vi "Reorder cluster elements v1.2.vi"(8 "error in (no error)":errorcluster, 10 "Reference Variant":variant, 11 "Data Variant":variant) -> (0 "error out":errorcluster, 1 "Reference key names":string[](array[string]), 2 "Ordered VCluster":variant, 3 "Queried key names":string[](array[string]))   [LabVIEW 2015]
uses:
  <vilib>/Utility/Data Type/NI_Data Type.lvlib
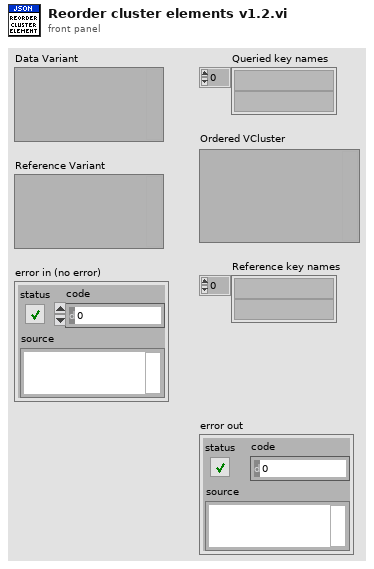
[diagram p1: front panel]
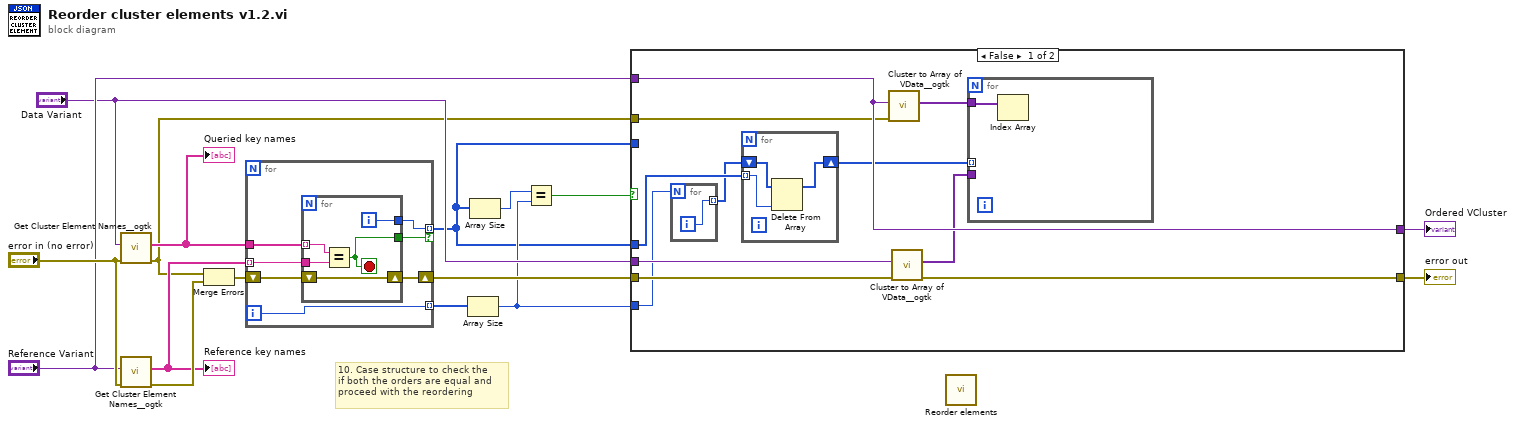
[diagram p0: block diagram]
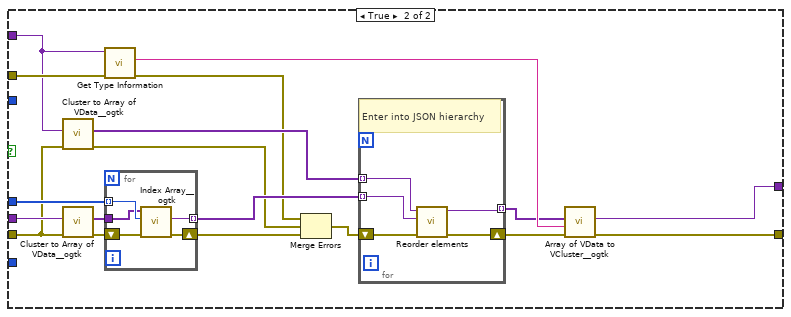
[diagram p2: hidden frame]
diagram:
  # "10. Case structure to check the\nif both the orders are equal and \nproceed with the reordering"
  n1 = call <userlib>:"Get Cluster Element Names__ogtk.vi"("error in (no error)"="error in (no error)", "Cluster"="Data Variant") -> ("error out"=w7:errorcluster, "Element Names"=w13:string[])  [unwired: 8 in]
  "Queried key names" <- w13
  n2 = call <userlib>:"Get Cluster Element Names__ogtk.vi"("error in (no error)"="error in (no error)", "Cluster"="Reference Variant") -> ("error out"=w14:errorcluster, "Element Names"=w12:string[])  [unwired: 8 in]
  "Reference key names" <- w12
  n3 = Merge Errors(w7, w14) -> (w15:errorcluster)
  n4 = for {
    tunnel: w12 -> [w22] mode=indexing
    tunnel: w13 -> [w23]
    tunnel: [w21] -> w1 mode=indexing if=w17
    shift-right: [w19] -> w16
    shift-left: w15 -> [w20]
    tunnel: [w18] -> w3 mode=indexing
    i -> [w18]
    n5 = for {
      tunnel: w23 -> [w28] mode=indexing
      tunnel: w22 -> [w27]
      tunnel: [w26] -> w21
      shift-right: [w25] -> w19
      shift-left: w20 -> [w25]
      tunnel: [w24] -> w17
      i -> [w26]
      stop <- w24 stop-if-true
      n6 = Equal?(x=w28, y=w27) -> (x = y?=w24:bool)
    }
  }
  n7 = Array Size(array=w3) -> (size(s)=w2:i32)
  n8 = Array Size(array=w1) -> (size(s)=w5:i32)
  n9 = Equal?(x=w5, y=w2) -> (x = y?=w4:bool)
  n10 = case shown="False" w4 {
    tunnel: w1 -> [w33 w62]
    tunnel: w16 -> [w36 w54]
    tunnel: "Reference Variant" -> [w37 w53]
    tunnel: "Data Variant" -> [w38 w59]
    tunnel: [w39 w49] -> w8
    tunnel: w7 -> [w35 w58]
    tunnel: [w37 w56] -> w6
    tunnel: w2 -> [w34 _]
    tunnel: w1 -> [_ _]
    frame False {
      n11 = for {
        N: w34 -> [_]
        tunnel: [w44] -> w32 mode=indexing
        i -> [w44]
      }
      n12 = for {
        tunnel: w33 -> [w42] mode=indexing
        shift-right: [w41] -> w31
        shift-left: w32 -> [w43]
        n13 = Delete From Array(array=w43, index=w42) -> (array with subset deleted=w41:i32[])  [unwired: 1 in, 1 out]
      }
      n14 = call <userlib>:"Cluster to Array of VData__ogtk.vi"("error in (no error)"=w35, "Cluster"=w37) -> ("Array of VData"=w29:variant[])  [unwired: 8 in, 1 out]
      n15 = call <userlib>:"Cluster to Array of VData__ogtk.vi"("error in (no error)"=w36, "Cluster"=w38) -> ("error out"=w39:errorcluster, "Array of VData"=w30:variant[])  [unwired: 8 in]
      n16 = for {
        tunnel: w31 -> [_] mode=indexing
        tunnel: w30 -> [_]
        tunnel: w29 -> [w40]
        n17 = Index Array(array=w40) -> ()  [unwired: 1 in, 1 out]
      }
    }
    frame True {
      n18 = call <userlib>:"Cluster to Array of VData__ogtk.vi"("error in (no error)"=w54, "Cluster"=w53) -> ("error out"=w46:errorcluster, "Array of VData"=w52:variant[])  [unwired: 8 in]
      n19 = call <userlib>:"Cluster to Array of VData__ogtk.vi"("error in (no error)"=w54, "Cluster"=w59) -> ("error out"=w61:errorcluster, "Array of VData"=w60:variant[])  [unwired: 8 in]
      n20 = call <vilib>:"Get Type Information.vi"("error in (no error)"=w58, "Variant"=w53) -> ("error out"=w45:errorcluster, "Name"=w48:string)  [unwired: 5 in, 3 out]
      n21 = for {
        tunnel: w60 -> [w68]
        shift-right: [w69] -> w57
        shift-left: w61 -> [w70]
        tunnel: w62 -> [w72] mode=indexing
        tunnel: [w71] -> w55 mode=indexing
        n22 = call <userlib>:"Index Array__ogtk.vi"("error in (no error)"=w70, "Index (1D)"=w72, "MultiD Array"=w68) -> ("error out"=w69:errorcluster, "Array Element"=w71:variant)  [unwired: 7 in]
      }
      n23 = Merge Errors(w45, w46, w57) -> (w51:errorcluster)
      n24 = for {
        shift-right: [w66] -> w50
        shift-left: w51 -> [w67]
        tunnel: w55 -> [w64] mode=indexing
        tunnel: w52 -> [w65] mode=indexing
        tunnel: [w63] -> w47 mode=indexing
        # "Enter into JSON hierarchy"
        n25 = call "Reorder elements.vi"("error in (no error)"=w67, "Data Variant"=w64, "Reference Variant"=w65) -> ("error out"=w66:errorcluster, "Output VData"=w63:variant)  [unwired: 7 in]
      }
      n26 = call <userlib>:"Array of VData to VCluster__ogtk.vi"("error in (no error)"=w50, "Cluster Name"=w48, "Array"=w47) -> ("error out"=w49:errorcluster, "VCluster"=w56:variant)  [unwired: 7 in]
    }
  }
  "error out" <- w8
  "Ordered VCluster" <- w6
  n27 = call "Reorder elements.vi"() -> ()  [unwired: 10 in, 2 out]
